vi "Fetch All Model Numbers.vi"(8 "error in (no error)":errorcluster, 11 "Database in":refnum<queue>) -> (0 "error out":errorcluster, 2 "Sensor Models":string[](array[string]), 3 "Database out":refnum<queue>)   [LabVIEW 2026]
uses:
  Architecture/Message Queue/Message Queue.lvlib
  Architecture/Message Queue/Enqueue Message (Single).vi
  Architecture/Message Queue/Message Cluster.ctl
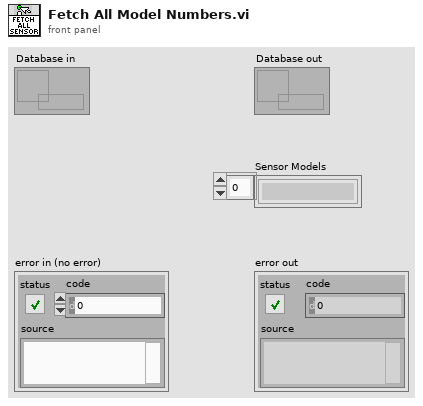
[diagram p1: front panel]
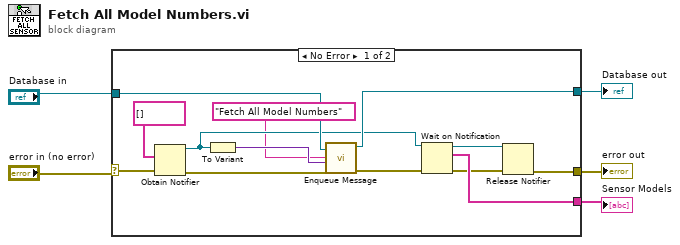
[diagram p0: block diagram]
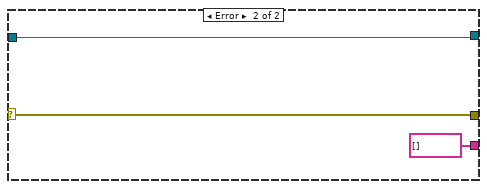
[diagram p2: hidden frame]
diagram:
  n1 = case shown="No Error" "error in (no error)" {
    selector: "error in (no error)" -> [w6 w20]
    tunnel: [w18 string[] []] -> w5
    tunnel: [w17 w21] -> w4
    tunnel: "Database in" -> [w16 w21]
    tunnel: [w15 w20] -> w2
    frame No Error {
      n2 = Obtain Notifier(notification data type=string[] [], error in (no error)=w6) -> (notifier out=w12:refnum<notifier>, error out=w9:errorcluster)  [unwired: 2 in, 1 out]
      n3 = To Variant(anything=w12) -> (Variant=w11:variant)
      n4 = call-poly "Enqueue Message.vi"("error in (no error)"=w9, "Message Data"=w11, "Message"="Fetch All Model Numbers", "Message Queue"=w16) -> ("error out"=w10:errorcluster, "dup Message Queue"=w17:refnum<queue>)  [unwired: 6 in]
      n5 = Wait on Notification(notifier=w12, error in (no error)=w10) -> (notifier out=w14:refnum<notifier>, notification=w18:string[], error out=w13:errorcluster)  [unwired: 2 in, 1 out]
      n6 = Release Notifier(notifier=w14, error in (no error)=w13) -> (error out=w15:errorcluster)  [unwired: 1 in, 2 out]
    }
    frame Error {
    }
  }
  "Sensor Models" <- w5
  "Database out" <- w4
  "error out" <- w2
